vi "AddIfTrue.vi"(9 "To Add":refnum<class "Action.lvclass">[](array[class]), 10 "True?":bool, 11 "Stack in":refnum<class "Stack.lvclass">) -> (3 "Stack out":refnum<class "Stack.lvclass">)   [LabVIEW 2024, in "ActionStack.lvlib" / "Stack.lvclass"]
uses:
  Stack.lvclass
  Action/Action.lvclass
  Stack.lvclass/Stack.ctl
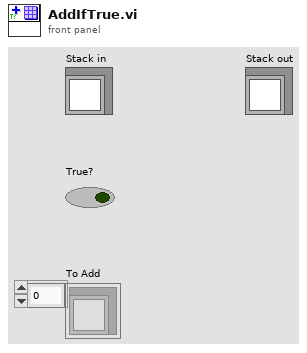
[diagram p1: front panel]
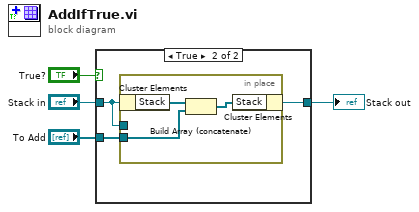
[diagram p0: block diagram]
diagram:
  n1 = case shown="True" "True?" {
    tunnel: [w5 w6] -> w4
    tunnel: "Stack in" -> [w5 w7]
    tunnel: "To Add" -> [_ w8]
    frame False {
    }
    frame True {
      n2 = in-place {
        in-place-border: w7 -> [_]
        in-place-border: w8 -> [w11]
        n3 = in-place-cluster #1(w7) -> ("Stack"=w10:refnum<class "Action.lvclass">[])
        n4 = Build Array (concatenate)(w10, w11) -> (w9:refnum<class "Action.lvclass">[])
        n5 = in-place-cluster #1("Stack"=w9) -> (w6:refnum<class "Stack.lvclass">)
      }
    }
  }
  "Stack out" <- w4
